vi "Validate Input Switch State.vi"(0 "VISA resource name":refnum<visa-resource-name>, 7 "Scan List (Empty: front panel)":string, 11 "error in (no error)":errorcluster) -> (4 "VISA resource name out":refnum<visa-resource-name>, 8 "Rear?":bool, 15 "error out":errorcluster)   [LabVIEW 2015, in "Keithley 27XX.lvlib"]
doc: "This VI queries and compares the state of the Front/Rear Input Switch to the Scan List. It returns an error if the Input Switch is not in the proper state, given the channels being scanned in the Scan List. For instance, if the Scan List is empty (front panel input), this VI will return an error if the Input Switch is not set to the \"Front\" state."
uses:
  Keithley 27XX.lvlib
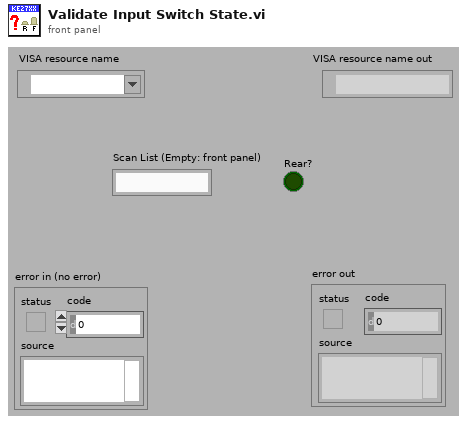
[diagram p1: front panel]
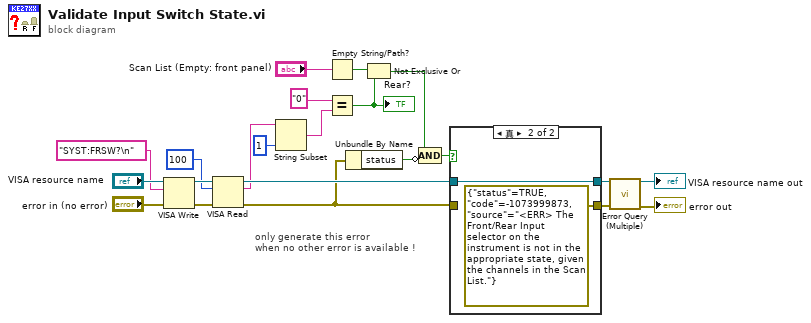
[diagram p0: block diagram]
diagram:
  # "only generate this error\nwhen no other error is available !"
  n1 = VISA Write(VISA resource name="VISA resource name", write buffer="SYST:FRSW?\n", error in (no error)="error in (no error)") -> (VISA resource name out=w17:refnum<visa-resource-name>, error out=w16:errorcluster)  [unwired: 1 out]
  n2 = VISA Read(VISA resource name=w17, byte count=u32 100, error in (no error)=w16) -> (VISA resource name out=w9:refnum<visa-resource-name>, read buffer=w7:string, error out=w4:errorcluster)  [unwired: 1 out]
  n3 = String Subset(string=w7, length (rest)=1 ("length (rest)")) -> (substring=w5:string)  [unwired: 1 in]
  n4 = Empty String/Path?(string/path="Scan List (Empty: front panel)") -> (empty?=w12:bool)
  n5 = Equal?(x="0", y=w5) -> (x = y?=w11:bool)
  "Rear?" <- w11
  n6 = Unbundle By Name(w4) -> ("status"=w3:bool)
  n7 = Not Exclusive Or(1:w11, 2:w12) -> (0:w2:bool)
  n8 = Compound Arithmetic op=AND(w2, invert w3) -> (w1:bool)
  n9 = case shown="真" w1 {
    tunnel: [w24 errorcluster {"status"=TRUE, "code"=-1073999873, "source"="<ERR> The Front/Rear Input selector on the instrument is not in the appropriate state, given the channels in the Scan List."} ("error out")] -> w10
    tunnel: w4 -> [w24 _]
    tunnel: w9 -> [w23 w25]
    tunnel: [w23 w25] -> w8
    frame False {
    }
    frame True {
    }
  }
  n10 = call "Error Query (Multiple).vi"("VISA resource name"=w8, "error in (no error)"=w10) -> ("VISA resource name out"=→"VISA resource name out":refnum<visa-resource-name>, "error out"=→"error out":errorcluster)  [unwired: 10 in, 2 out]
